vi "Write.vi"(0 "GenericCanAdapterClass in":refnum<class "GenericCanAdapterClass.lvclass">, 5 "Id":u32 format="%08x", 7 "DataLength":i32, 9 "Data":u8[](array[numeric]) format="%02x", 11 "error in (no error)":errorcluster) -> (4 "GenericCanAdapterClass out":refnum<class "GenericCanAdapterClass.lvclass">, 15 "error out":errorcluster)   [LabVIEW 2011, in "GenericCanAdapterClass.lvclass"]
uses:
  GenericCanAdapterClass.lvclass
  Private/LogCanTxMessage.vi
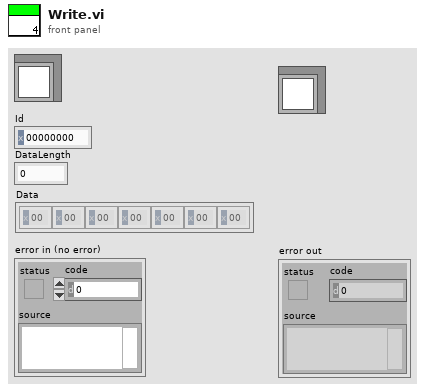
[diagram p1: front panel]
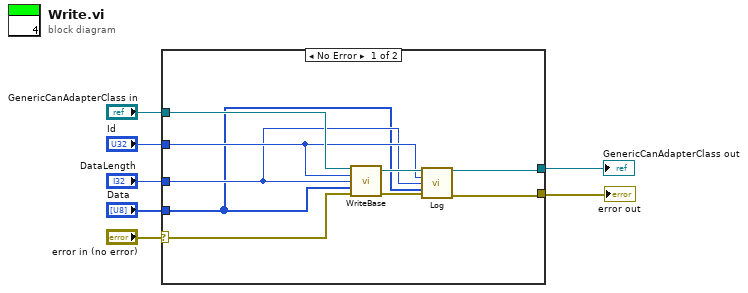
[diagram p0: block diagram]
diagram:
  n1 = case shown="No Error" "error in (no error)" {
    selector: "error in (no error)" -> [w15 w18]
    tunnel: [w13 w18] -> w6
    tunnel: [w12 w17] -> w4
    tunnel: "GenericCanAdapterClass in" -> [w16 w17]
    tunnel: "Id" -> [w10 _]
    tunnel: "DataLength" -> [w9 _]
    tunnel: "Data" -> [w8 _]
    frame No Error {
      n2 = call-dynamic "WriteBase.vi"("GenericCanAdapterClass in"=w16, "Id"=w10, "DataLength"=w9, "Data"=w8, "error in (no error)"=w15) -> ("GenericCanAdapterClass out"=w11:refnum<class "GenericCanAdapterClass.lvclass">, "error out"=w14:errorcluster)  [unwired: 9 in]
      n3 = call-poly "Log.vi"("GenericCanAdapterClass in"=w11, "Arbitration Id"=w10, "DataLength"=w9, "Data"=w8, "error in"=w14) -> ("GenericCanAdapterClass out"=w12:refnum<class "GenericCanAdapterClass.lvclass">, "error out"=w13:errorcluster)  [unwired: 9 in]
    }
    frame Error {
    }
  }
  "error out" <- w6
  "GenericCanAdapterClass out" <- w4
